vi "FTW-Endpoint-Core-Receive.vi"(0 "FTW Endpoint":refnum<class "FTW-Endpoint.lvclass">, 5 "Timeout":i32 format="%dmsec", 11 "error in":errorcluster) -> (4 "FTW Endpoint out":refnum<class "FTW-Endpoint.lvclass">, 6 "Message":string, 8 "Message Received?":bool, 13 "Message Length":u64, 14 "Message Pointer":i64, 15 "error out":errorcluster)   [LabVIEW 2012, in "FTW-Actor.lvlib" / "FTW-Endpoint.lvclass"]
uses:
  FTW-Endpoint.lvclass
  FTW-Endpoint.lvclass/FTW-Endpoint.ctl
panel:
  out "Message Length 2":u64
  out "Message Pointer 2":i64
  # "Inputs"
  # "Outputs"
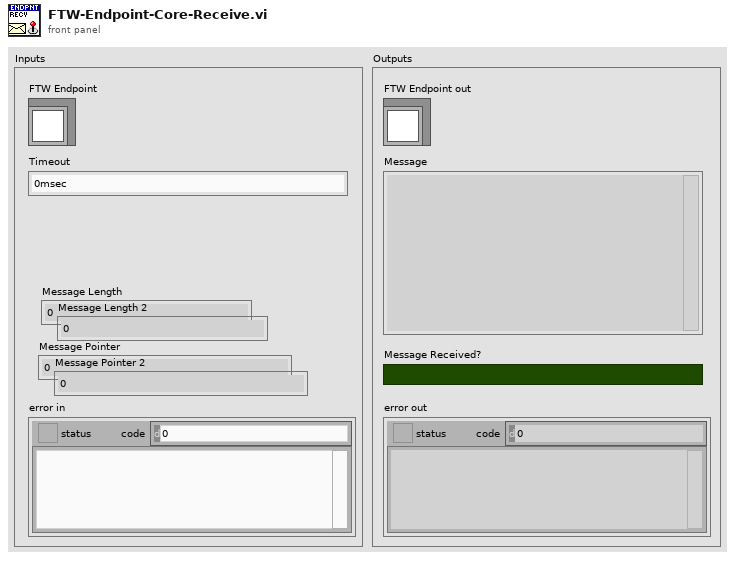
[diagram p1: front panel]
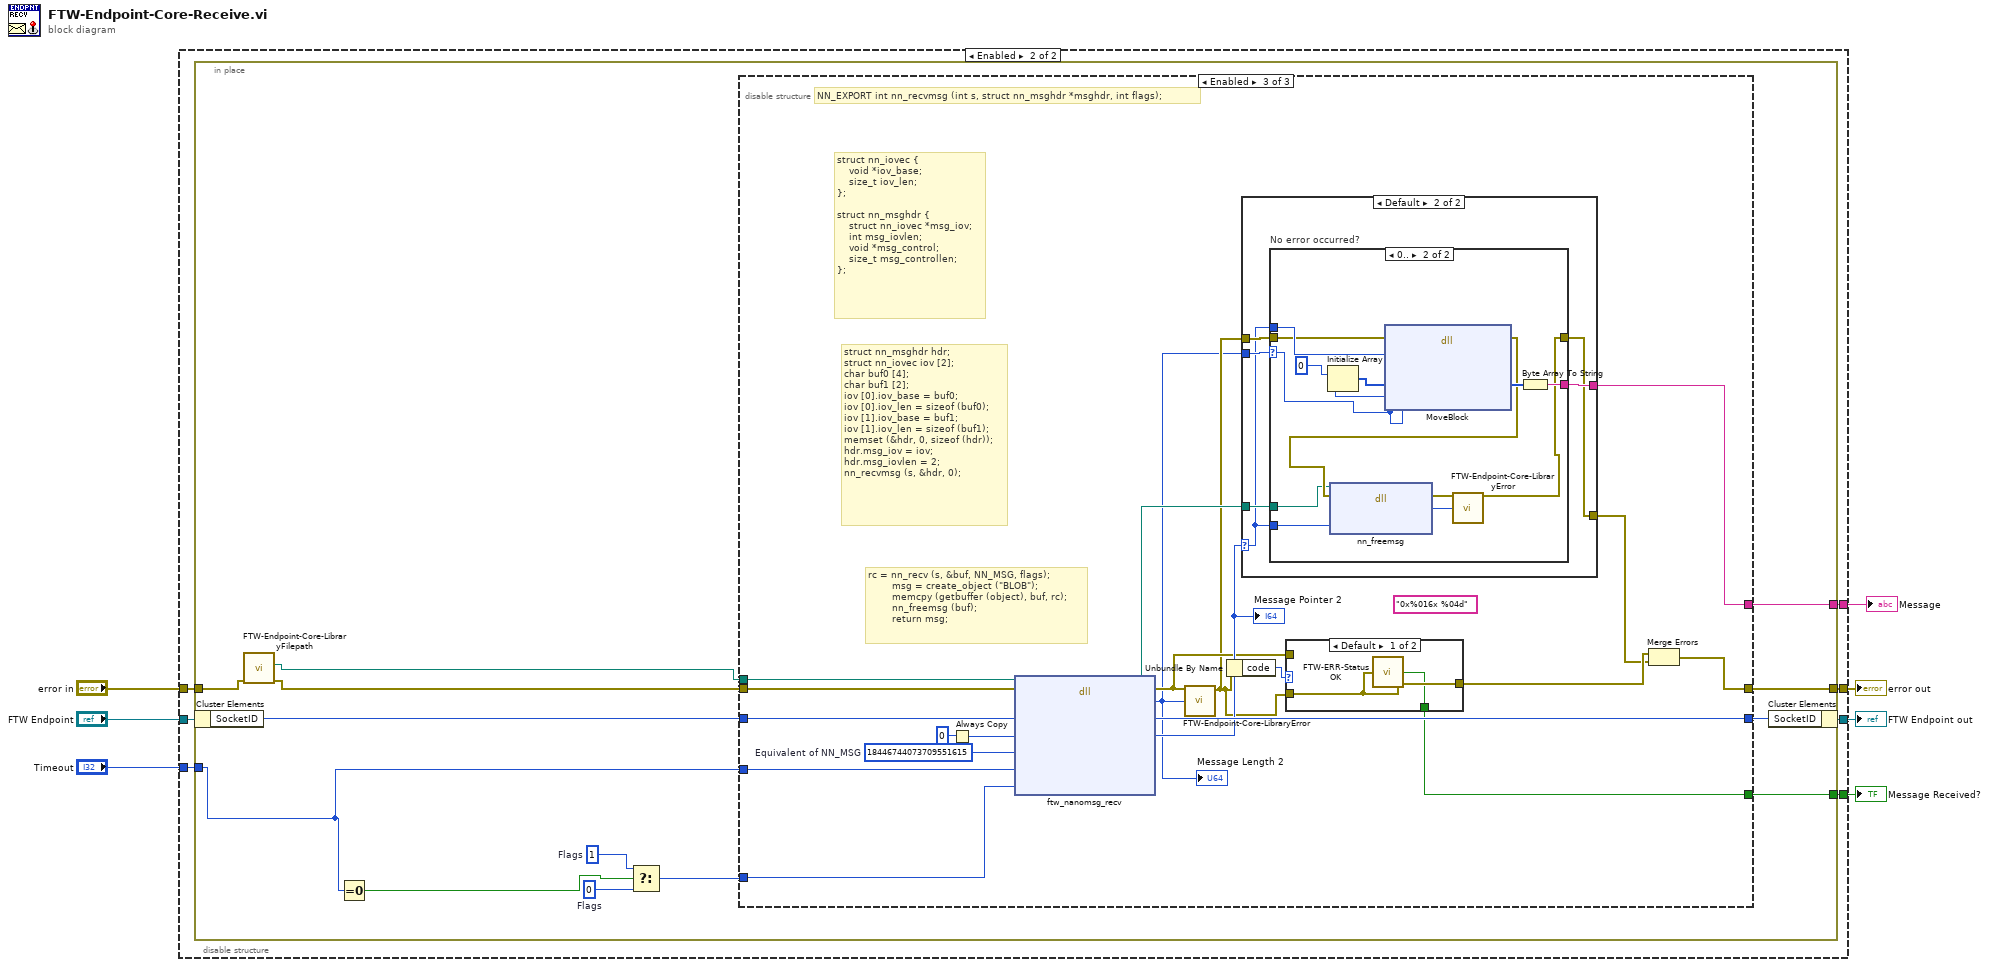
[diagram p0: block diagram]
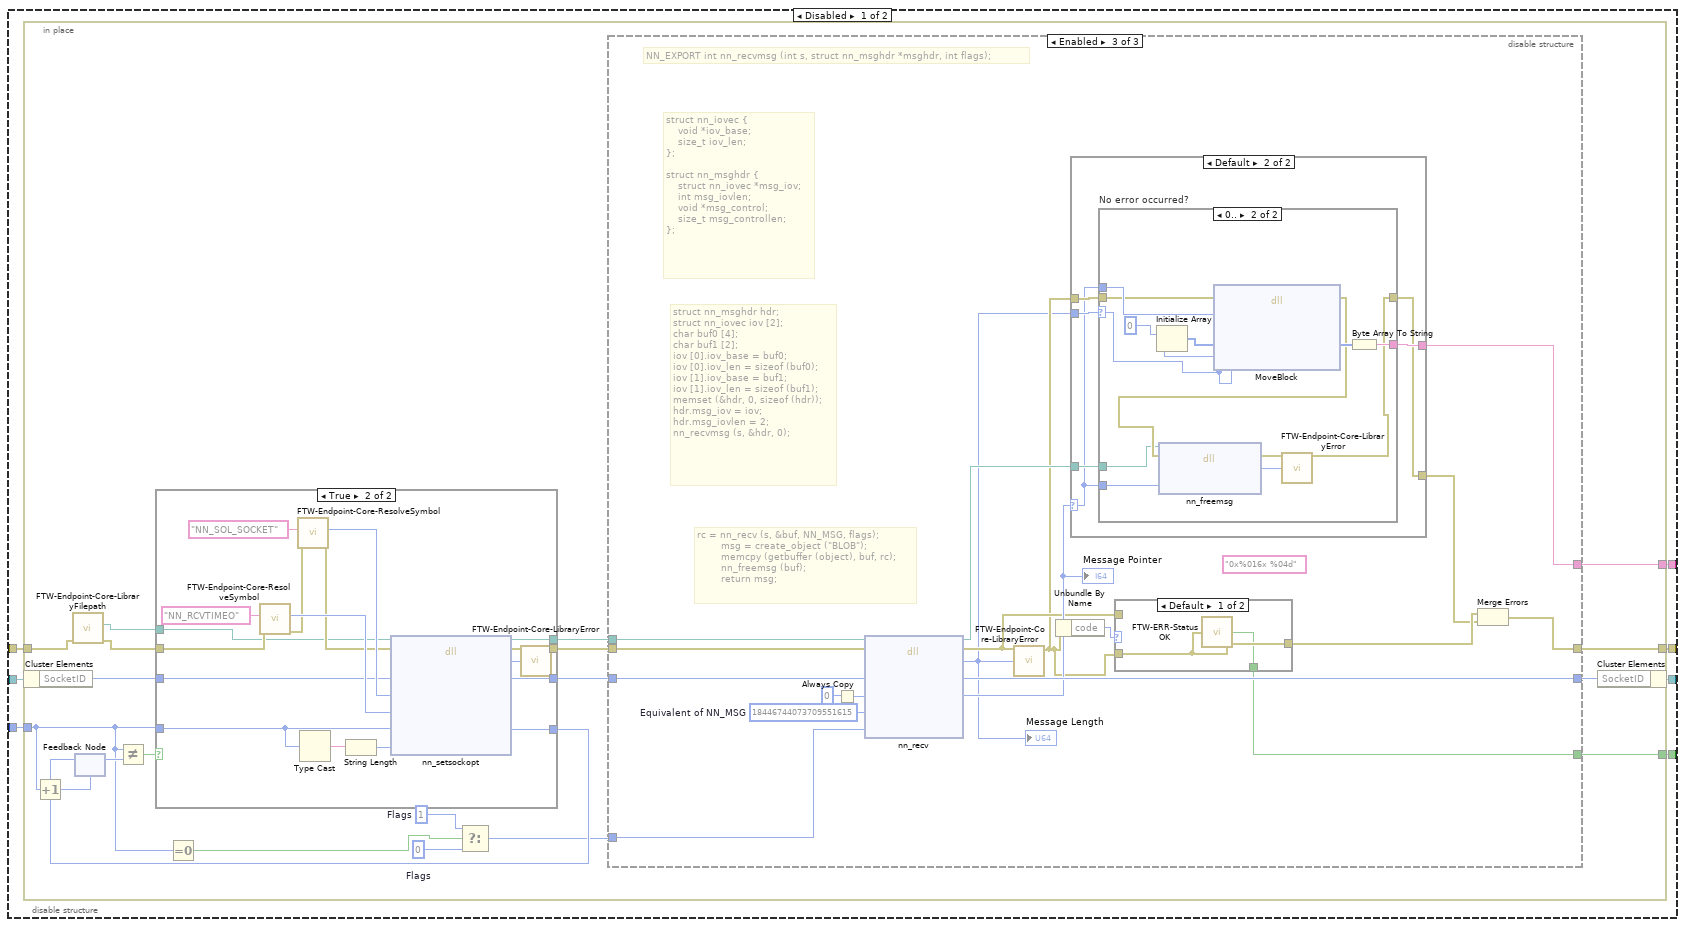
[diagram p2: hidden frame]
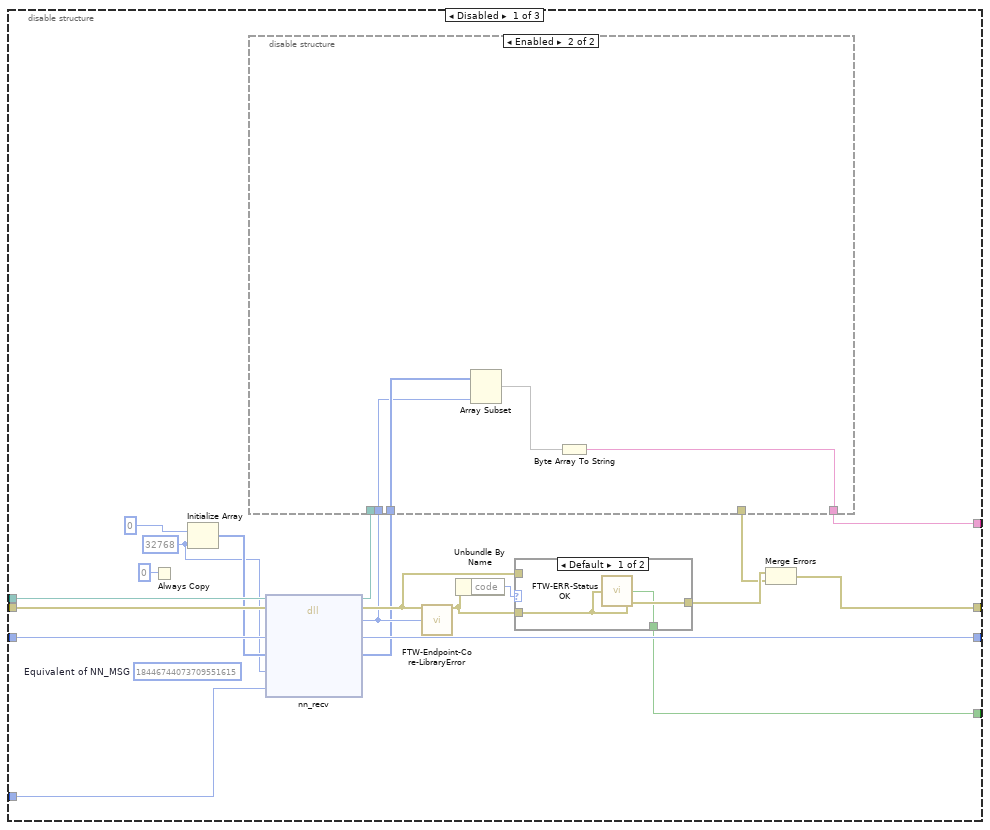
[diagram p3: hidden frame]
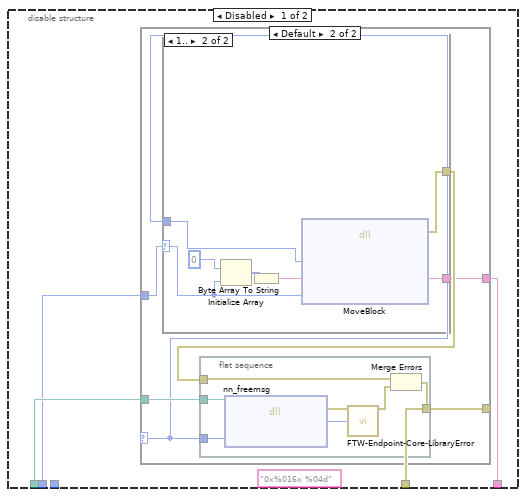
[diagram p4: hidden frame]
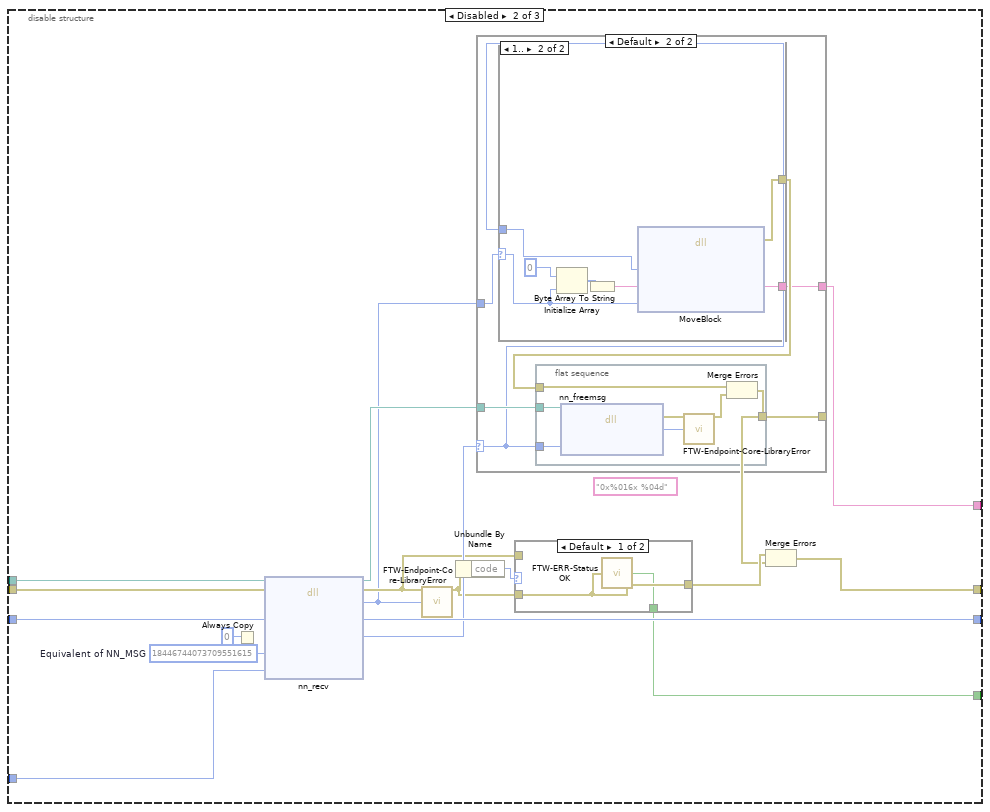
[diagram p8: hidden frame]
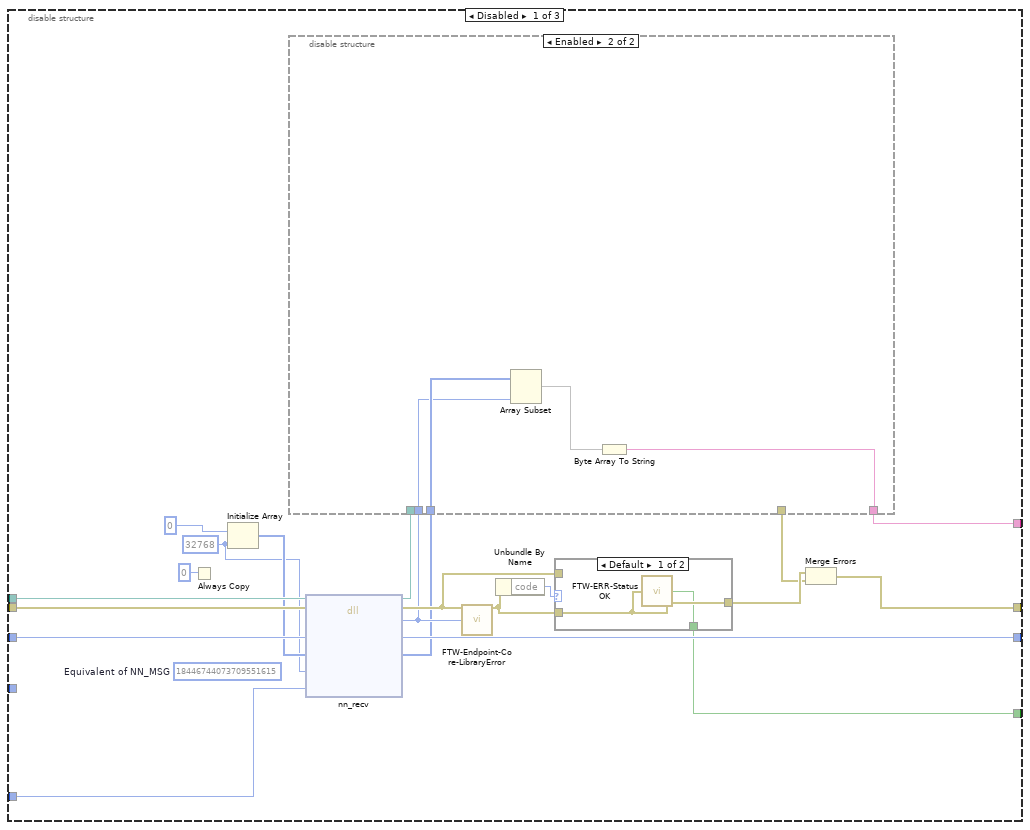
[diagram p16: hidden frame]
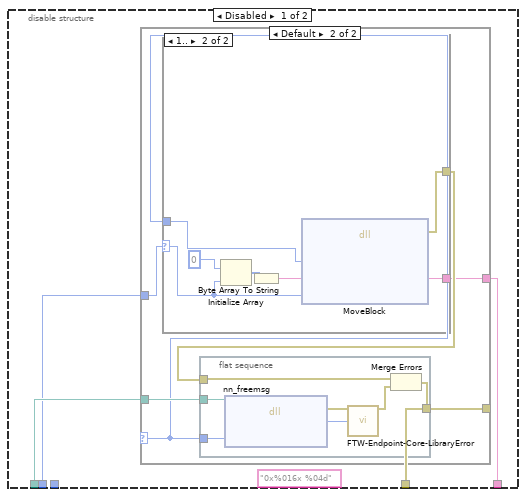
[diagram p17: hidden frame]
diagram:
  n1 = disable-structure shown="Enabled" {
    disable-tunnel: "error in" -> [w14 w198]
    disable-tunnel: [w13 w197] -> w6
    disable-tunnel: "FTW Endpoint" -> [w12 w196]
    disable-tunnel: [w11 w195] -> w4
    disable-tunnel: [w10 w194] -> w3
    disable-tunnel: "Timeout" -> [w9 w193]
    disable-tunnel: [w8 w192] -> w1
    frame Disabled {
      n2 = in-place {
        in-place-border: w14 -> [w25]
        in-place-border: [w29] -> w13
        in-place-border: [w22] -> w10
        in-place-border: w9 -> [w16]
        in-place-border: [w18] -> w8
        w20 = 0  # Flags
        w21 = 1  # Flags
        n3 = in-place-cluster #1(w12) -> ("SocketID"=w33:i64)
        n4 = Increment(x=w16) -> (x+1=w17:i32)
        n5 = call "FTW-Endpoint-Core-LibraryFilepath.vi"("error in"=w25) -> ("error out"=w24:errorcluster, "Library Filepath"=w23:path)  [unwired: 8 in, 1 out]
        n6 = feedback #2(w17) -> (w28:i32)
        n7 = Not Equal?(x=w16, y=w28) -> (x != y?=w26:bool)
        n8 = case shown="True" w26 {
          tunnel: w24 -> [w173 w175]
          tunnel: w33 -> [w172 w184]
          tunnel: [w172 w183] -> w32
          tunnel: [w173 w181] -> w31
          tunnel: [w170 w180] -> w30
          tunnel: w16 -> [w171 w177]
          tunnel: [w171 w176] -> w27
          tunnel: w23 -> [w170 w174]
          frame False {
          }
          frame True {
            n9 = call "FTW-Endpoint-Core-ResolveSymbol.vi"("error in"=w175, "Symbol"="NN_RCVTIMEO") -> ("error out"=w185:errorcluster, "Symbol Value"=w188:i32)  [unwired: 8 in]
            n10 = call "FTW-Endpoint-Core-ResolveSymbol.vi"("error in"=w185, "Symbol"="NN_SOL_SOCKET") -> ("error out"=w182:errorcluster, "Symbol Value"=w186:i32)  [unwired: 8 in]
            n11 = Type Cast(x=w177) -> (*(type *) &x=w179:string)  [unwired: 1 in]
            n12 = String Length(string=w179) -> (length=w178:i32)
            n13 = dll-call lib="?" fn="nn_setsockopt"(path in=w174, error in=w182, "SocketID"=w184, "Option Level"=w186, "Option"=w188, "Option Value"=w177, "Option Value Length"=w178) -> (path out=w180:path, error out=w190:errorcluster, "Return Value"=w191:i64, "SocketID"=w183:i64, "Option Value"=w176:i32)  [unwired: 4 in]
            n14 = call "FTW-Endpoint-Core-LibraryError.vi"("error in"=w190, "Return Value"=w191) -> ("error out"=w181:errorcluster)  [unwired: 13 in]
          }
        }
        n15 = feedback-in #2(w27) -> ()
        n16 = Equal To 0?(x=w16) -> (x = 0?=w15:bool)
        n17 = Select(t=w21, s=w15, f=w20) -> (s? t:f=w19:i32)
        n18 = disable-structure shown="Enabled" {
          disable-tunnel: [w54 w103 w145] -> w34
          disable-tunnel: w32 -> [w52 w100 w143]
          disable-tunnel: w31 -> [w51 w99 w142]
          disable-tunnel: w30 -> [w50 w98 w141]
          disable-tunnel: [w45 w92 w137] -> w29
          disable-tunnel: [w41 w88 w135] -> w22
          disable-tunnel: w19 -> [w40 w87 w134]
          disable-tunnel: [w39 w86 w133] -> w18
          frame Disabled {
            w35 = 32768 ("dimension size")
            (unwired) u64 18446744073709551615  # Equivalent of NN_MSG
            n19 = Always Copy(1:i64 0 ("buf")) -> ()  [unwired: 1 out]
            n20 = Initialize Array(u8 0 ("element"), w35) -> (w36:u8[])
            n21 = dll-call lib="?" fn="nn_recv"(path in=w50, error in=w51, "SocketID"=w52, "Message Buffer"=w36, "Message Length"=w35, "Flags"=w40) -> (path out=w53:path, error out=w43:errorcluster, "Return Value"=w42:i64, "SocketID"=w54:i64, "Message Buffer"=w38:u8[])  [unwired: 3 in]
            n22 = disable-structure shown="Enabled" {
              disable-tunnel: w53 -> [w58 _]
              disable-tunnel: [w57 _] -> w44
              disable-tunnel: w42 -> [w56 w80]
              disable-tunnel: [w55 w82] -> w41
              disable-tunnel: w38 -> [_ w81]
              frame Disabled {
                (unwired) "0x%016x %04d" ("format string")
                n23 = case shown="Default" {
                  selector: _ -> [_ w59]
                  tunnel: [_ w64] -> w57
                  tunnel: w58 -> [_ w63]
                  tunnel: w56 -> [_ w61]
                  tunnel: [_ w60] -> w55
                  frame 0 {
                  }
                  frame Default {
                    n24 = case shown="1.." w61 {
                      selector: w61 -> [_ w69]
                      tunnel: [_ w66] -> w62
                      tunnel: [_ w65] -> w60
                      tunnel: w59 -> [_ w71]
                      frame ..0 {
                      }
                      frame 1.. {
                        n25 = Initialize Array(u8 0, w69) -> (w68:u8[])
                        n26 = Byte Array To String(unsigned byte array=w68) -> (string=w67:string)
                        n27 = dll-call lib="LabVIEW" fn="MoveBlock"("Source Pointer"=w71, "Pointer to Destination"=w67, "String Length"=w69) -> (error out=w66:errorcluster, "Pointer to Destination"=w65:string)  [unwired: 6 in, 1 out]
                      }
                    }
                    n28 = flat-sequence {
                      tunnel: [w72] -> w64
                      tunnel: w63 -> [w76]
                      tunnel: w59 -> [w75]
                      tunnel: w62 -> [w73]
                      frame #0 {
                        n29 = dll-call lib="?" fn="nn_freemsg"(path in=w76, "Message Pointer"=w75) -> (error out=w78:errorcluster, "Return Value"=w77:i64)  [unwired: 3 in, 1 out]
                        n30 = call "FTW-Endpoint-Core-LibraryError.vi"("error in"=w78, "Return Value"=w77) -> ("error out"=w74:errorcluster)  [unwired: 13 in]
                        n31 = Merge Errors(w73, w74) -> (w72:errorcluster)
                      }
                    }
                  }
                }
              }
              frame Enabled {
                n32 = Array Subset(array=w81, length=w80) -> (w79:u8[])  [unwired: 1 in]
                n33 = Byte Array To String(unsigned byte array=w79) -> (string=w82:string)
              }
            }
            n34 = call "FTW-Endpoint-Core-LibraryError.vi"("error in"=w43, "Return Value"=w42) -> ("error out"=w47:errorcluster)  [unwired: 13 in]
            n35 = Unbundle By Name(w47) -> ("code"=w48:i32)
            n36 = case shown="Default" w48 {
              tunnel: [w84 w85] -> w46
              tunnel: w47 -> [w84 _]
              tunnel: w43 -> [_ w85]
              tunnel: [w83 _] -> w39
              frame Default {
                n37 = call "FTW-ERR-StatusOK.vi"("error to check"=w84) -> ("Status OK?"=w83:bool)
              }
              frame 11 {
              }
            }
            n38 = Merge Errors(w46, w44) -> (w45:errorcluster)
          }
          frame Disabled {
            (unwired) "0x%016x %04d" ("format string")
            w102 = u64 18446744073709551615  # Equivalent of NN_MSG
            n39 = Always Copy(1:i64 0 ("buf")) -> ()  [unwired: 1 out]
            n40 = dll-call lib="?" fn="nn_recv"(path in=w98, error in=w99, "SocketID"=w100, "Message Length"=w102, "Flags"=w87) -> (path out=w101:path, error out=w90:errorcluster, "Return Value"=w89:i64, "SocketID"=w103:i64, "Message Pointer"=w96:i64)  [unwired: 4 in]
            n41 = call "FTW-Endpoint-Core-LibraryError.vi"("error in"=w90, "Return Value"=w89) -> ("error out"=w94:errorcluster)  [unwired: 13 in]
            n42 = Unbundle By Name(w94) -> ("code"=w95:i32)
            n43 = case shown="Default" w96 {
              selector: w96 -> [_ w104]
              tunnel: [_ w109] -> w91
              tunnel: w101 -> [_ w108]
              tunnel: w89 -> [_ w106]
              tunnel: [_ w105] -> w88
              frame 0 {
              }
              frame Default {
                n44 = case shown="1.." w106 {
                  selector: w106 -> [_ w114]
                  tunnel: [_ w111] -> w107
                  tunnel: [_ w110] -> w105
                  tunnel: w104 -> [_ w116]
                  frame ..0 {
                  }
                  frame 1.. {
                    n45 = Initialize Array(u8 0, w114) -> (w113:u8[])
                    n46 = Byte Array To String(unsigned byte array=w113) -> (string=w112:string)
                    n47 = dll-call lib="LabVIEW" fn="MoveBlock"("Source Pointer"=w116, "Pointer to Destination"=w112, "String Length"=w114) -> (error out=w111:errorcluster, "Pointer to Destination"=w110:string)  [unwired: 6 in, 1 out]
                  }
                }
                n48 = flat-sequence {
                  tunnel: [w117] -> w109
                  tunnel: w108 -> [w121]
                  tunnel: w104 -> [w120]
                  tunnel: w107 -> [w118]
                  frame #0 {
                    n49 = dll-call lib="?" fn="nn_freemsg"(path in=w121, "Message Pointer"=w120) -> (error out=w123:errorcluster, "Return Value"=w122:i64)  [unwired: 3 in, 1 out]
                    n50 = call "FTW-Endpoint-Core-LibraryError.vi"("error in"=w123, "Return Value"=w122) -> ("error out"=w119:errorcluster)  [unwired: 13 in]
                    n51 = Merge Errors(w118, w119) -> (w117:errorcluster)
                  }
                }
              }
            }
            n52 = case shown="Default" w95 {
              tunnel: [w125 w126] -> w93
              tunnel: w94 -> [w125 _]
              tunnel: w90 -> [_ w126]
              tunnel: [w124 _] -> w86
              frame Default {
                n53 = call "FTW-ERR-StatusOK.vi"("error to check"=w125) -> ("Status OK?"=w124:bool)
              }
              frame 11 {
              }
            }
            n54 = Merge Errors(w93, w91) -> (w92:errorcluster)
          }
          frame Enabled {
            (unwired) "0x%016x %04d" ("format string")
            w144 = u64 18446744073709551615  # Equivalent of NN_MSG
            # "struct nn_msghdr hdr;\nstruct nn_iovec iov [2];\nchar buf0 [4];\nchar buf1 [2];\niov [0].iov_base = buf0;\niov [0].iov_len = sizeof (buf0);\niov [1].iov_base = buf1;\niov [1].iov_len = sizeof (buf1);\nmemset (&hdr, 0, sizeof (hdr));\nhdr.msg_iov = iov;\nhdr.msg_iovlen = 2;\nnn_recvmsg (s, &hdr, 0);"
            # "struct nn_iovec {\n    void *iov_base;\n    size_t iov_len;\n};\n\nstruct nn_msghdr {\n    struct nn_iovec *msg_iov;\n    int msg_iovlen;\n    void *msg_control;\n    size_t msg_controllen;\n};"
            # "NN_EXPORT int nn_recvmsg (int s, struct nn_msghdr *msghdr, int flags);"
            # "rc = nn_recv (s, &buf, NN_MSG, flags);\n        msg = create_object (\"BLOB\");\n        memcpy (getbuffer (object), buf, rc);\n        nn_freemsg (buf);\n        return msg;"
            n55 = Always Copy(1:i64 0 ("buf")) -> (0:w127:i64)
            n56 = dll-call lib="?" fn="nn_recv"(path in=w141, error in=w142, "SocketID"=w143, "Message Pointer"=w127, "Message Length"=w144, "Flags"=w134) -> (path out=w132:path, error out=w130:errorcluster, "Return Value"=w128:i64, "SocketID"=w145:i64, "Message Pointer"=w131:i64)  [unwired: 3 in]
            "Message Length" <- w128
            "Message Pointer" <- w131
            n57 = call "FTW-Endpoint-Core-LibraryError.vi"("error in"=w130, "Return Value"=w128) -> ("error out"=w129:errorcluster)  [unwired: 13 in]
            n58 = Unbundle By Name(w129) -> ("code"=w139:i32)
            n59 = case shown="Default" w131 {
              selector: w131 -> [_ w147]
              tunnel: [w146 w149] -> w136
              tunnel: w132 -> [_ w148]
              tunnel: w128 -> [_ w152]
              tunnel: [_ w151] -> w135
              tunnel: w129 -> [w146 w150]
              frame 0 {
              }
              frame Default {
                n60 = case "No error occurred?" shown="0.." w152 {
                  selector: w152 -> [_ w160]
                  tunnel: [w153 w154] -> w149
                  tunnel: [_ w161] -> w151
                  tunnel: w147 -> [_ w166]
                  tunnel: w150 -> [w153 w164]
                  tunnel: w148 -> [_ w158]
                  tunnel: w147 -> [_ w157]
                  frame ..-1 {
                  }
                  frame 0.. {
                    n61 = Initialize Array(u8 0, w160) -> (w163:u8[])
                    n62 = dll-call lib="LabVIEW" fn="MoveBlock"(error in=w164, "Source Pointer"=w166, "Pointer to Destination"=w163, "String Length"=w160) -> (error out=w159:errorcluster, "Pointer to Destination"=w162:u8[])  [unwired: 5 in, 1 out]
                    n63 = dll-call lib="?" fn="nn_freemsg"(path in=w158, error in=w159, "Message Pointer"=w157) -> (error out=w156:errorcluster, "Return Value"=w155:i64)  [unwired: 2 in, 1 out]
                    n64 = call "FTW-Endpoint-Core-LibraryError.vi"("error in"=w156, "Return Value"=w155) -> ("error out"=w154:errorcluster)  [unwired: 13 in]
                    n65 = Byte Array To String(unsigned byte array=w162) -> (string=w161:string)
                  }
                }
              }
            }
            n66 = case shown="Default" w139 {
              tunnel: [w168 w169] -> w138
              tunnel: w129 -> [w168 _]
              tunnel: w130 -> [_ w169]
              tunnel: [w167 _] -> w133
              frame Default {
                n67 = call "FTW-ERR-StatusOK.vi"("error to check"=w168) -> ("Status OK?"=w167:bool)
              }
              frame 11 {
              }
            }
            n68 = Merge Errors(w138, w136) -> (w137:errorcluster)
          }
        }
        n69 = in-place-cluster #1("SocketID"=w34) -> (w11:refnum<class "FTW-Endpoint.lvclass">)
      }
    }
    frame Enabled {
      n70 = in-place {
        in-place-border: w198 -> [w209]
        in-place-border: [w210] -> w197
        in-place-border: [w208] -> w194
        in-place-border: w193 -> [w199]
        in-place-border: [w204] -> w192
        w206 = 0  # Flags
        w207 = 1  # Flags
        n71 = in-place-cluster #3(w196) -> ("SocketID"=w202:i64)
        n72 = call "FTW-Endpoint-Core-LibraryFilepath.vi"("error in"=w209) -> ("error out"=w201:errorcluster, "Library Filepath"=w200:path)  [unwired: 8 in, 1 out]
        n73 = Equal To 0?(x=w199) -> (x = 0?=w203:bool)
        n74 = Select(t=w207, s=w203, f=w206) -> (s? t:f=w205:i32)
        n75 = disable-structure shown="Enabled" {
          disable-tunnel: [w231 w280 w323] -> w211
          disable-tunnel: w202 -> [w229 w277 w321]
          disable-tunnel: w201 -> [w228 w276 w320]
          disable-tunnel: w200 -> [w227 w275 w319]
          disable-tunnel: [w222 w269 w315] -> w210
          disable-tunnel: [w218 w265 w313] -> w208
          disable-tunnel: w205 -> [w217 w264 w312]
          disable-tunnel: [w216 w263 w311] -> w204
          disable-tunnel: w199 -> [_ _ w304]
          frame Disabled {
            w212 = 32768 ("dimension size")
            (unwired) u64 18446744073709551615  # Equivalent of NN_MSG
            n76 = Always Copy(1:i64 0 ("buf")) -> ()  [unwired: 1 out]
            n77 = Initialize Array(u8 0 ("element"), w212) -> (w213:u8[])
            n78 = dll-call lib="?" fn="nn_recv"(path in=w227, error in=w228, "SocketID"=w229, "Message Buffer"=w213, "Message Length"=w212, "Flags"=w217) -> (path out=w230:path, error out=w220:errorcluster, "Return Value"=w219:i64, "SocketID"=w231:i64, "Message Buffer"=w215:u8[])  [unwired: 3 in]
            n79 = disable-structure shown="Enabled" {
              disable-tunnel: w230 -> [w235 _]
              disable-tunnel: [w234 _] -> w221
              disable-tunnel: w219 -> [w233 w257]
              disable-tunnel: [w232 w259] -> w218
              disable-tunnel: w215 -> [_ w258]
              frame Disabled {
                (unwired) "0x%016x %04d" ("format string")
                n80 = case shown="Default" {
                  selector: _ -> [_ w236]
                  tunnel: [_ w241] -> w234
                  tunnel: w235 -> [_ w240]
                  tunnel: w233 -> [_ w238]
                  tunnel: [_ w237] -> w232
                  frame 0 {
                  }
                  frame Default {
                    n81 = case shown="1.." w238 {
                      selector: w238 -> [_ w246]
                      tunnel: [_ w243] -> w239
                      tunnel: [_ w242] -> w237
                      tunnel: w236 -> [_ w248]
                      frame ..0 {
                      }
                      frame 1.. {
                        n82 = Initialize Array(u8 0, w246) -> (w245:u8[])
                        n83 = Byte Array To String(unsigned byte array=w245) -> (string=w244:string)
                        n84 = dll-call lib="LabVIEW" fn="MoveBlock"("Source Pointer"=w248, "Pointer to Destination"=w244, "String Length"=w246) -> (error out=w243:errorcluster, "Pointer to Destination"=w242:string)  [unwired: 6 in, 1 out]
                      }
                    }
                    n85 = flat-sequence {
                      tunnel: [w249] -> w241
                      tunnel: w240 -> [w253]
                      tunnel: w236 -> [w252]
                      tunnel: w239 -> [w250]
                      frame #0 {
                        n86 = dll-call lib="?" fn="nn_freemsg"(path in=w253, "Message Pointer"=w252) -> (error out=w255:errorcluster, "Return Value"=w254:i64)  [unwired: 3 in, 1 out]
                        n87 = call "FTW-Endpoint-Core-LibraryError.vi"("error in"=w255, "Return Value"=w254) -> ("error out"=w251:errorcluster)  [unwired: 13 in]
                        n88 = Merge Errors(w250, w251) -> (w249:errorcluster)
                      }
                    }
                  }
                }
              }
              frame Enabled {
                n89 = Array Subset(array=w258, length=w257) -> (w256:u8[])  [unwired: 1 in]
                n90 = Byte Array To String(unsigned byte array=w256) -> (string=w259:string)
              }
            }
            n91 = call "FTW-Endpoint-Core-LibraryError.vi"("error in"=w220, "Return Value"=w219) -> ("error out"=w224:errorcluster)  [unwired: 13 in]
            n92 = Unbundle By Name(w224) -> ("code"=w225:i32)
            n93 = case shown="Default" w225 {
              tunnel: [w261 w262] -> w223
              tunnel: w224 -> [w261 _]
              tunnel: w220 -> [_ w262]
              tunnel: [w260 _] -> w216
              frame Default {
                n94 = call "FTW-ERR-StatusOK.vi"("error to check"=w261) -> ("Status OK?"=w260:bool)
              }
              frame 11 {
              }
            }
            n95 = Merge Errors(w223, w221) -> (w222:errorcluster)
          }
          frame Disabled {
            (unwired) "0x%016x %04d" ("format string")
            w279 = u64 18446744073709551615  # Equivalent of NN_MSG
            n96 = Always Copy(1:i64 0 ("buf")) -> ()  [unwired: 1 out]
            n97 = dll-call lib="?" fn="nn_recv"(path in=w275, error in=w276, "SocketID"=w277, "Message Length"=w279, "Flags"=w264) -> (path out=w278:path, error out=w267:errorcluster, "Return Value"=w266:i64, "SocketID"=w280:i64, "Message Pointer"=w273:i64)  [unwired: 4 in]
            n98 = call "FTW-Endpoint-Core-LibraryError.vi"("error in"=w267, "Return Value"=w266) -> ("error out"=w271:errorcluster)  [unwired: 13 in]
            n99 = Unbundle By Name(w271) -> ("code"=w272:i32)
            n100 = case shown="Default" w273 {
              selector: w273 -> [_ w281]
              tunnel: [_ w286] -> w268
              tunnel: w278 -> [_ w285]
              tunnel: w266 -> [_ w283]
              tunnel: [_ w282] -> w265
              frame 0 {
              }
              frame Default {
                n101 = case shown="1.." w283 {
                  selector: w283 -> [_ w291]
                  tunnel: [_ w288] -> w284
                  tunnel: [_ w287] -> w282
                  tunnel: w281 -> [_ w293]
                  frame ..0 {
                  }
                  frame 1.. {
                    n102 = Initialize Array(u8 0, w291) -> (w290:u8[])
                    n103 = Byte Array To String(unsigned byte array=w290) -> (string=w289:string)
                    n104 = dll-call lib="LabVIEW" fn="MoveBlock"("Source Pointer"=w293, "Pointer to Destination"=w289, "String Length"=w291) -> (error out=w288:errorcluster, "Pointer to Destination"=w287:string)  [unwired: 6 in, 1 out]
                  }
                }
                n105 = flat-sequence {
                  tunnel: [w294] -> w286
                  tunnel: w285 -> [w298]
                  tunnel: w281 -> [w297]
                  tunnel: w284 -> [w295]
                  frame #0 {
                    n106 = dll-call lib="?" fn="nn_freemsg"(path in=w298, "Message Pointer"=w297) -> (error out=w300:errorcluster, "Return Value"=w299:i64)  [unwired: 3 in, 1 out]
                    n107 = call "FTW-Endpoint-Core-LibraryError.vi"("error in"=w300, "Return Value"=w299) -> ("error out"=w296:errorcluster)  [unwired: 13 in]
                    n108 = Merge Errors(w295, w296) -> (w294:errorcluster)
                  }
                }
              }
            }
            n109 = case shown="Default" w272 {
              tunnel: [w302 w303] -> w270
              tunnel: w271 -> [w302 _]
              tunnel: w267 -> [_ w303]
              tunnel: [w301 _] -> w263
              frame Default {
                n110 = call "FTW-ERR-StatusOK.vi"("error to check"=w302) -> ("Status OK?"=w301:bool)
              }
              frame 11 {
              }
            }
            n111 = Merge Errors(w270, w268) -> (w269:errorcluster)
          }
          frame Enabled {
            (unwired) "0x%016x %04d" ("format string")
            w322 = u64 18446744073709551615  # Equivalent of NN_MSG
            # "struct nn_msghdr hdr;\nstruct nn_iovec iov [2];\nchar buf0 [4];\nchar buf1 [2];\niov [0].iov_base = buf0;\niov [0].iov_len = sizeof (buf0);\niov [1].iov_base = buf1;\niov [1].iov_len = sizeof (buf1);\nmemset (&hdr, 0, sizeof (hdr));\nhdr.msg_iov = iov;\nhdr.msg_iovlen = 2;\nnn_recvmsg (s, &hdr, 0);"
            # "struct nn_iovec {\n    void *iov_base;\n    size_t iov_len;\n};\n\nstruct nn_msghdr {\n    struct nn_iovec *msg_iov;\n    int msg_iovlen;\n    void *msg_control;\n    size_t msg_controllen;\n};"
            # "NN_EXPORT int nn_recvmsg (int s, struct nn_msghdr *msghdr, int flags);"
            # "rc = nn_recv (s, &buf, NN_MSG, flags);\n        msg = create_object (\"BLOB\");\n        memcpy (getbuffer (object), buf, rc);\n        nn_freemsg (buf);\n        return msg;"
            n112 = Always Copy(1:i64 0 ("buf")) -> (0:w305:i64)
            n113 = dll-call lib="?" fn="ftw_nanomsg_recv"(path in=w319, error in=w320, "SocketID"=w321, "Message Pointer"=w305, "Message Length"=w322, "Timeout"=w304, "Flags"=w312) -> (path out=w310:path, error out=w308:errorcluster, "Return Value"=w306:i64, "SocketID"=w323:i64, "Message Pointer"=w309:i64)  [unwired: 4 in]
            "Message Length 2" <- w306
            "Message Pointer 2" <- w309
            n114 = call "FTW-Endpoint-Core-LibraryError.vi"("error in"=w308, "Return Value"=w306) -> ("error out"=w307:errorcluster)  [unwired: 13 in]
            n115 = Unbundle By Name(w307) -> ("code"=w317:i32)
            n116 = case shown="Default" w309 {
              selector: w309 -> [_ w325]
              tunnel: [w324 w327] -> w314
              tunnel: w310 -> [_ w326]
              tunnel: w306 -> [_ w330]
              tunnel: [_ w329] -> w313
              tunnel: w307 -> [w324 w328]
              frame 0 {
              }
              frame Default {
                n117 = case "No error occurred?" shown="0.." w330 {
                  selector: w330 -> [_ w338]
                  tunnel: [w331 w332] -> w327
                  tunnel: [_ w339] -> w329
                  tunnel: w325 -> [_ w344]
                  tunnel: w328 -> [w331 w342]
                  tunnel: w326 -> [_ w336]
                  tunnel: w325 -> [_ w335]
                  frame ..-1 {
                  }
                  frame 0.. {
                    n118 = Initialize Array(u8 0, w338) -> (w341:u8[])
                    n119 = dll-call lib="LabVIEW" fn="MoveBlock"(error in=w342, "Source Pointer"=w344, "Pointer to Destination"=w341, "String Length"=w338) -> (error out=w337:errorcluster, "Pointer to Destination"=w340:u8[])  [unwired: 5 in, 1 out]
                    n120 = dll-call lib="?" fn="nn_freemsg"(path in=w336, error in=w337, "Message Pointer"=w335) -> (error out=w334:errorcluster, "Return Value"=w333:i64)  [unwired: 2 in, 1 out]
                    n121 = call "FTW-Endpoint-Core-LibraryError.vi"("error in"=w334, "Return Value"=w333) -> ("error out"=w332:errorcluster)  [unwired: 13 in]
                    n122 = Byte Array To String(unsigned byte array=w340) -> (string=w339:string)
                  }
                }
              }
            }
            n123 = case shown="Default" w317 {
              tunnel: [w346 w347] -> w316
              tunnel: w307 -> [w346 _]
              tunnel: w308 -> [_ w347]
              tunnel: [w345 _] -> w311
              frame Default {
                n124 = call "FTW-ERR-StatusOK.vi"("error to check"=w346) -> ("Status OK?"=w345:bool)
              }
              frame 11 {
              }
            }
            n125 = Merge Errors(w316, w314) -> (w315:errorcluster)
          }
        }
        n126 = in-place-cluster #3("SocketID"=w211) -> (w195:refnum<class "FTW-Endpoint.lvclass">)
      }
    }
  }
  "error out" <- w6
  "FTW Endpoint out" <- w4
  "Message Received?" <- w1
  "Message" <- w3
